vi "close.vi"(8 "error in (no error)":errorcluster, 11 "Telnet in":refnum<class "Telnet.lvclass">) -> (0 "error out":errorcluster, 3 "Telnet out":refnum<class "Telnet.lvclass">)   [LabVIEW 2011, in "Hardware.lvlib" / "HWControllers.lvlib" / "Telnet.lvclass"]
uses:
  Telnet.lvclass
  Telnet.lvclass/Telnet.ctl
  <vilib>/addons/internet/NI_InternetTK_Core_VIs.lvlib
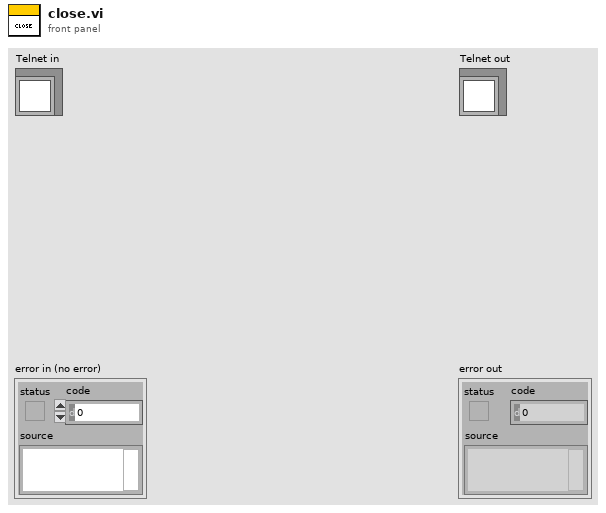
[diagram p1: front panel]
types:
  T1 = typedef "Telnet Session.ctl" = refnum<k1>
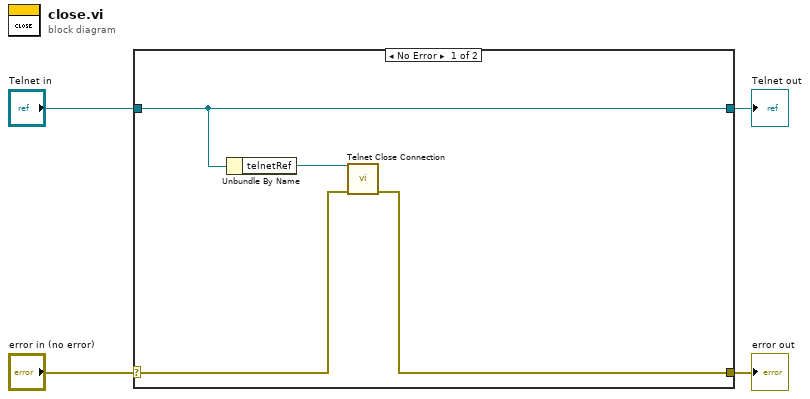
[diagram p0: block diagram]
diagram:
  n1 = case shown="No Error" "error in (no error)" {
    selector: "error in (no error)" -> [w6 w10]
    tunnel: [w5 w10] -> w3
    tunnel: [w8 w9] -> w1
    tunnel: "Telnet in" -> [w8 w9]
    frame No Error {
      n2 = Unbundle By Name(w8) -> ("telnetRef"=w7:T1)
      n3 = call <vilib>:"Telnet Close Connection.vi"("error in (no error)"=w6, "telnet connection"=w7) -> ("error out"=w5:errorcluster)  [unwired: 8 in, 1 out]
    }
    frame Error {
    }
  }
  "error out" <- w3
  "Telnet out" <- w1
